vi "Launcher.vi"(8 "error in (no error)":errorcluster, 11 "Process in":refnum<class "Process.lvclass">) -> (0 "error out":errorcluster, 3 "Process out":refnum<class "Process.lvclass">)   [LabVIEW 2019, in "TimingDRV Engine.lvlib" / "Process.lvclass"]
uses:
  Process.lvclass
  2291a6ca-4cbd-4d19-aa3f-3e1ab23b1054.vi
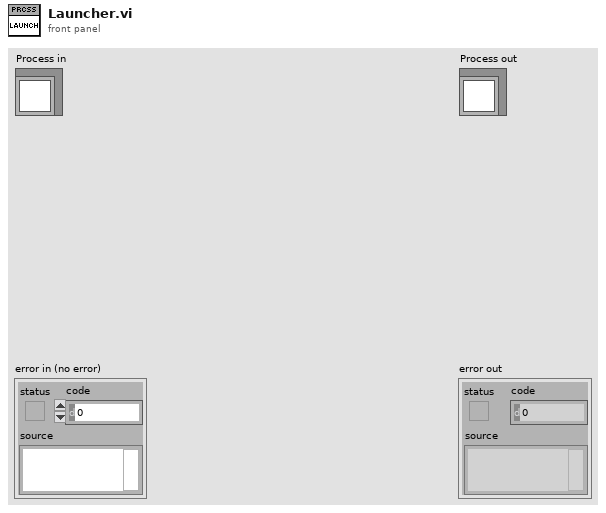
[diagram p1: front panel]
types:
  T1 = enum32{"invalid scope", "public", "private", "protected", "community"}
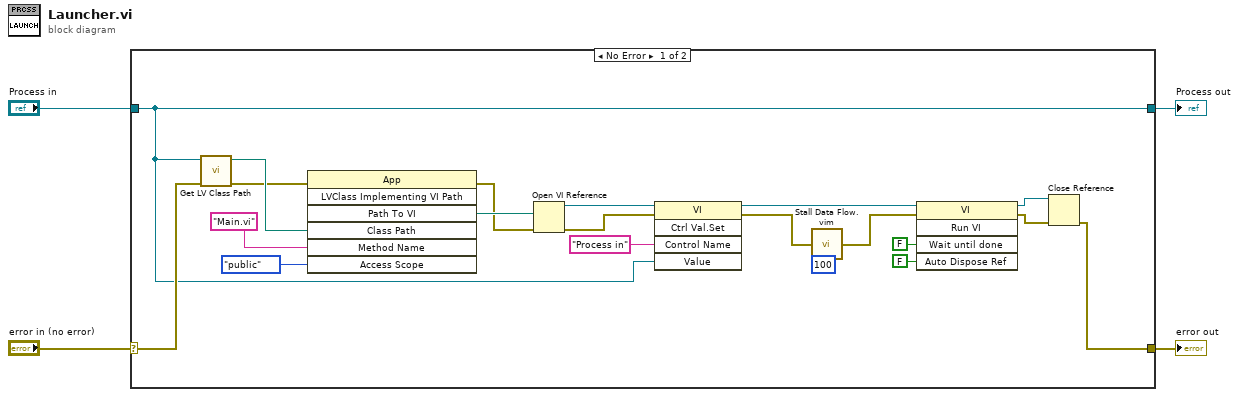
[diagram p0: block diagram]
diagram:
  n1 = case shown="No Error" "error in (no error)" {
    selector: "error in (no error)" -> [w24 w26]
    tunnel: [w18 w26] -> w3
    tunnel: [w14 w25] -> w1
    tunnel: "Process in" -> [w14 w25]
    frame No Error {
      n2 = call <vilib>:"Get LV Class Path.vi"("error in (no error)"=w24, "object"=w14) -> ("error out"=w21:errorcluster, "class path"=w23:path)  [unwired: 8 in]
      n3 = invoke class="App" method="LVClass Implementing VI Path"(error in=w21, "Class Path"=w23, "Method Name"="Main.vi", "Access Scope"=T1."public") -> (error out=w19:errorcluster, "Path To VI"=w20:path)  [unwired: 3 in, 5 out]
      n4 = Open VI Reference(vi path=w20, error in (no error)=w19) -> (vi reference=w17:refnum<vi>, error out=w16:errorcluster)  [unwired: 4 in]
      n5 = invoke class="VI" method="Ctrl Val.Set"(reference=w17, error in=w16, "Control Name"="Process in", "Value"=w14) -> (reference out=w5:refnum<vi>, error out=w7:errorcluster)  [unwired: 1 in, 3 out]
      n6 = call "Stall Data Flow.vim"("value in"=w7, "milliseconds to wait"=u32 100) -> ("value out"=w6:errorcluster)  [unwired: 1 out]
      n7 = invoke class="VI" method="Run VI"(reference=w5, error in=w6, "Wait until done"=FALSE ("Wait Until Done"), "Auto Dispose Ref"=FALSE ("Auto Dispose Reference")) -> (reference out=w11:refnum<vi>, error out=w8:errorcluster)  [unwired: 1 in, 3 out]
      n8 = Close Reference(reference=w11, error in (no error)=w8) -> (error out=w18:errorcluster)
    }
    frame Error {
    }
  }
  "error out" <- w3
  "Process out" <- w1
